vi "DisconnectK.vi"(0 "Keyence":T2={"Serial port sem"=refnum, "Serial port handle"="", "Baud rate"=9600}, 5 "error in":errorcluster) -> (19 "error out":errorcluster)   [LabVIEW 2018]
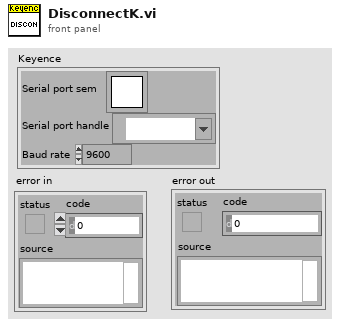
[diagram p1: front panel]
types:
  T1 = typedef "Semaphore RefNum" = refnum<k1>
  T2 = cluster{"Serial port sem":T1, "Serial port handle":refnum<visa-resource-name>, "Baud rate":u32}
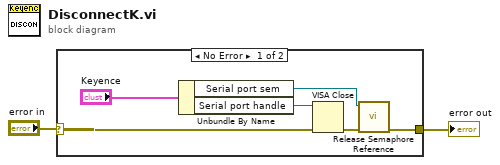
[diagram p0: block diagram]
diagram:
  n1 = case shown="No Error" "error in" {
    selector: "error in" -> [w8 w9]
    tunnel: [w6 w9] -> w1
    frame No Error {
      n2 = Unbundle By Name("Keyence") -> ("Serial port sem"=w5:T1, "Serial port handle"=w4:refnum<visa-resource-name>)
      n3 = VISA Close(VISA resource name=w4, error in (no error)=w8) -> (error out=w7:errorcluster)
      n4 = call <vilib>:"Release Semaphore Reference.vi"("error in (no error)"=w7, "semaphore"=w5) -> ("error out"=w6:errorcluster)  [unwired: 8 in, 1 out]
    }
    frame Error {
    }
  }
  "error out" <- w1
